vi "FP_Get Monitor WorkSpace.vi"(11 "Monitor Select":T4) -> (2 "Index Out":i32, 3 "Selected Work Space Out":T1, 5 "All Work Spaces Out":T3, 7 "Display:Primary Workspace Out":T2)   [LabVIEW 2025]
uses:
  TypeDefs_Utility/ENUM_Monitor Select.ctl
  <vilib>/Utility/miscctls.llb/LVAllMonitorsDisplayTypeDef.ctl
  <vilib>/Utility/miscctls.llb/LVRectTypeDef.ctl
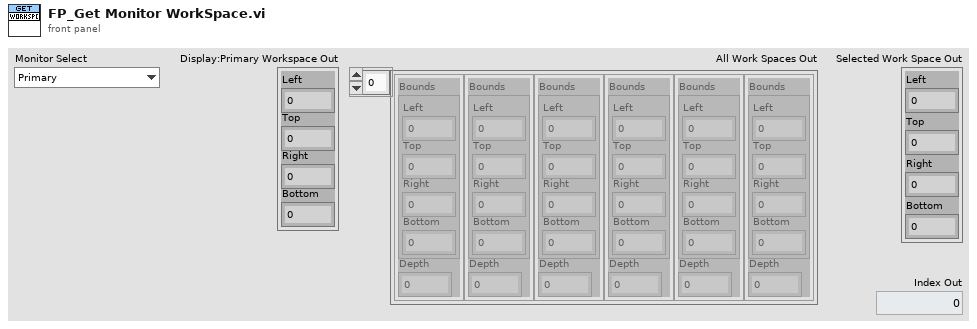
[diagram p1: front panel]
types:
  T1 = cluster{"Left":i16, "Top":i16, "Right":i16, "Bottom":i16}
  T2 = typedef "LVRectTypeDef.ctl" = cluster{"Left":i16, "Top":i16, "Right":i16, "Bottom":i16}
  T3 = typedef "LVAllMonitorsDisplayTypeDef.ctl" = cluster{"Bounds":cluster{"Left":i16, "Top":i16, "Right":i16, "Bottom":i16}, "Depth":i16}[]
  T4 = typedef "ENUM_Monitor Select.ctl" = enum16{"Primary", "Secondary (Right first)", "Right of Primary", "Left of Primary", "Above Primary", "Below Primary"}
  T5 = cluster{"Bounds":cluster{"Left":i16, "Top":i16, "Right":i16, "Bottom":i16}, "Depth":i16}
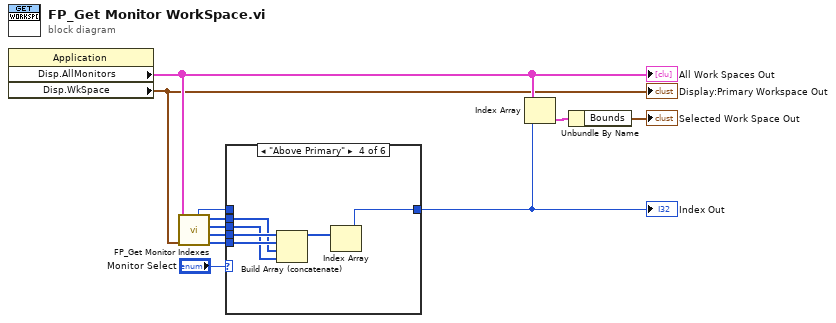
[diagram p0: block diagram]
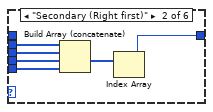
[diagram p3: hidden frame]
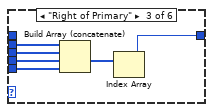
[diagram p4: hidden frame]
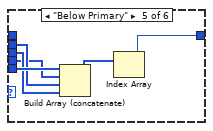
[diagram p5: hidden frame]
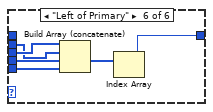
[diagram p6: hidden frame]
diagram:
  n1 = property class="Application"() -> ("Disp.AllMonitors"=w2:T3, "Disp.WkSpace"=w1:T2)  [unwired: 2 in, 2 out]
  "All Work Spaces Out" <- w2
  "Display:Primary Workspace Out" <- w1
  n2 = call "FP_Get Monitor Indexes.vi"("Primary"=w1, "All Work Spaces"=w2) -> ("Indexes Below Out"=w6:i32[], "Indexes Above Out"=w7:i32[], "Indexes Left Out"=w8:i32[], "Indexes Right Out"=w9:i32[], "Primary Index Out"=w10:i32)  [unwired: 5 in]
  n3 = case shown="\"Above Primary\"" "Monitor Select" {
    tunnel: w10 -> [w12 _ _ _ _ _]
    tunnel: w9 -> [_ w18 w24 w26 w33 w37]
    tunnel: w8 -> [_ w17 w23 w25 w32 w38]
    tunnel: w7 -> [_ w16 w22 w30 w31 w42]
    tunnel: w6 -> [_ w15 w21 w29 w34 w41]
    tunnel: [w12 w13 w19 w27 w35 w39] -> w4
    frame "Primary" {
    }
    frame "Secondary (Right first)" {
      n4 = Build Array (concatenate)(w18, w17, w16, w15) -> (w14:i32[])
      n5 = Index Array(array=w14) -> (element=w13:i32)  [unwired: 1 in]
    }
    frame "Right of Primary" {
      n6 = Build Array (concatenate)(w24, w23, w22, w21) -> (w20:i32[])
      n7 = Index Array(array=w20) -> (element=w19:i32)  [unwired: 1 in]
    }
    frame "Above Primary" {
      n8 = Build Array (concatenate)(w30, w29, w26, w25) -> (w28:i32[])
      n9 = Index Array(array=w28) -> (element=w27:i32)  [unwired: 1 in]
    }
    frame "Below Primary" {
      n10 = Build Array (concatenate)(w34, w31, w33, w32) -> (w36:i32[])
      n11 = Index Array(array=w36) -> (element=w35:i32)  [unwired: 1 in]
    }
    frame "Left of Primary" {
      n12 = Build Array (concatenate)(w38, w37, w42, w41) -> (w40:i32[])
      n13 = Index Array(array=w40) -> (element=w39:i32)  [unwired: 1 in]
    }
  }
  "Index Out" <- w4
  n14 = Index Array(array=w2, index=w4) -> (element=w5:T5)
  n15 = Unbundle By Name(w5) -> ("Bounds"=→"Selected Work Space Out":T1)
